vi "Write Results.lvclass.vi"(8 "error in (no error)":errorcluster, 10 "Results.lvclass":refnum<class "Results.lvclass">, 11 "Display Results in":refnum<class "Display Results.lvclass">) -> (0 "error out":errorcluster, 3 "Display Results out":refnum<class "Display Results.lvclass">)   [LabVIEW 2017, in "Measurement UI.lvlib" / "Display Results.lvclass"]
uses:
  Display Results.lvclass
  Results/Results.lvclass
  Display Results.lvclass/Display Results.ctl
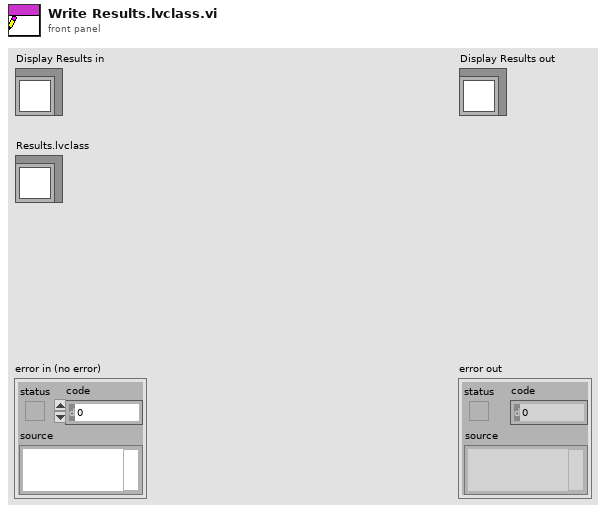
[diagram p1: front panel]
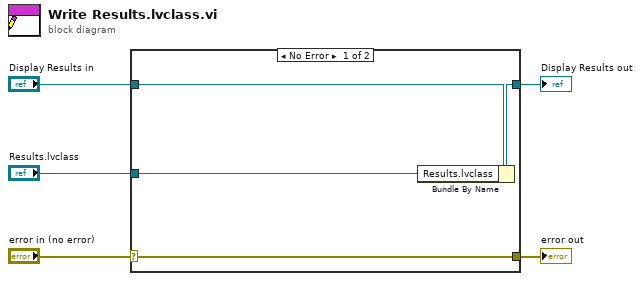
[diagram p0: block diagram]
diagram:
  n1 = case shown="No Error" "error in (no error)" {
    selector: "error in (no error)" -> [w9 w10]
    tunnel: [w9 w10] -> w4
    tunnel: [w7 w11] -> w2
    tunnel: "Display Results in" -> [w8 w11]
    tunnel: "Results.lvclass" -> [w6 _]
    frame No Error {
      n2 = Bundle By Name(cluster=w8, "Results.lvclass"=w6) -> (w7:refnum<class "Display Results.lvclass">)
    }
    frame Error {
    }
  }
  "error out" <- w4
  "Display Results out" <- w2
